vi "time_minfirstlast.vi"(3 "Sec. from Midnight":dbl) -> (0 "First Minute of Day":bool, 1 "Last Minute of Day":bool)   [LabVIEW 2018]
doc: "From the current time (in seconds from midnight, GMT), this VI determines whether the current time is within the first minute or last minute of the day."
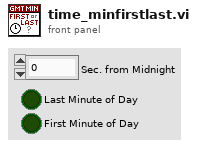
[diagram p1: front panel]
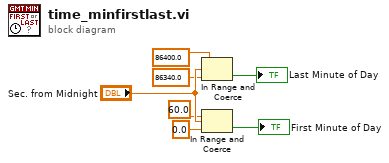
[diagram p0: block diagram]
diagram:
  n1 = In Range and Coerce(upper limit=86400.0, x="Sec. from Midnight", lower limit=86340.0) -> (In Range?=→"Last Minute of Day":bool)  [unwired: 1 out]
  n2 = In Range and Coerce(upper limit=60.0, x="Sec. from Midnight", lower limit=0.0) -> (In Range?=→"First Minute of Day":bool)  [unwired: 1 out]
